vi "Make from Input.vi"(8 "error in (no error)":errorcluster, 10 "Input":string) -> (0 "error out":errorcluster, 3 "Galaxy out":refnum<class "Galaxy.lvclass">[](array[class]))   [LabVIEW 2020, in "Galaxy.lvclass"]
uses:
  Galaxy.lvclass
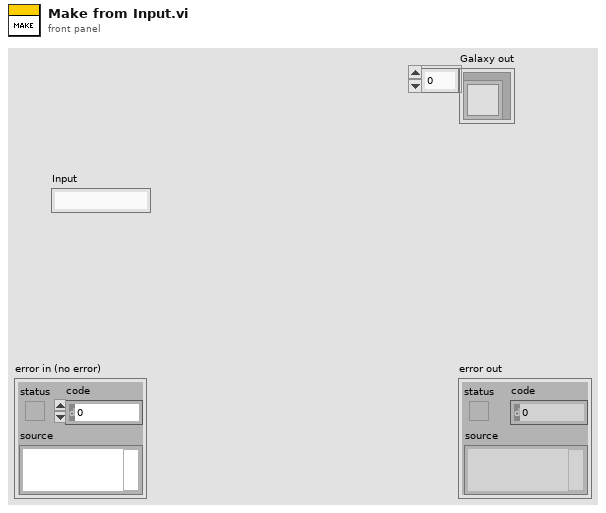
[diagram p1: front panel]
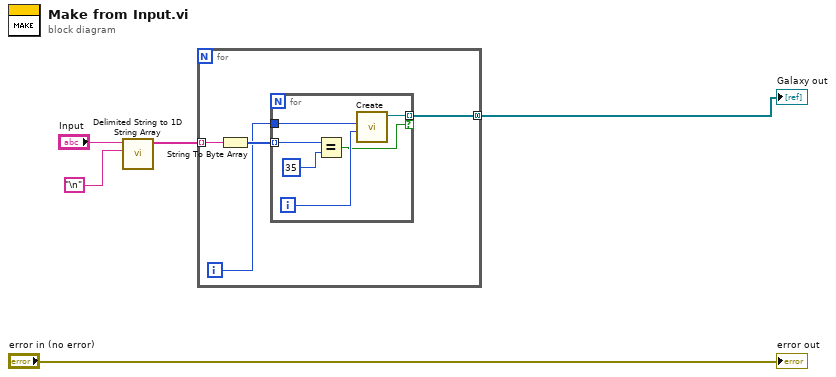
[diagram p0: block diagram]
diagram:
  n1 = call <vilib>:"Delimited String to 1D String Array.vi"("delimiter"="\n", "delimited string"="Input") -> ("string array"=w2:string[])  [unwired: 9 in]
  n2 = for {
    tunnel: w2 -> [w9] mode=indexing
    tunnel: [w6] -> w1 mode=concatenating
    i -> [w7]
    n3 = String To Byte Array(string=w9) -> (unsigned byte array=w8:u8[])
    n4 = for {
      tunnel: w8 -> [w15] mode=indexing
      tunnel: w7 -> [w12]
      tunnel: [w11] -> w6 mode=indexing if=w10
      i -> [w13]
      n5 = Equal?(x=w15, y=u8 35) -> (x = y?=w10:bool)
      n6 = call "Create.vi"("Col"=w13, "Row"=w12) -> ("Galaxy"=w11:refnum<class "Galaxy.lvclass">)  [unwired: 8 in, 1 out]
    }
  }
  "Galaxy out" <- w1
  "error out" <- "error in (no error)"
